vi "Test Remove.vi"() -> ()   [LabVIEW 2021, in "d15.lvlib" / "Cave.lvclass"]
uses:
  Cave.lvclass
  Diamond/Diamond.lvclass
panel:
  in  "Test":T1(ring)=enum."D in C"
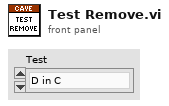
[diagram p1: front panel]
types:
  T1 = enum16{"D[1,2] in C", "D[1] in C", "D in C", "C[1,2] in D", "C in D", "D not in C"}
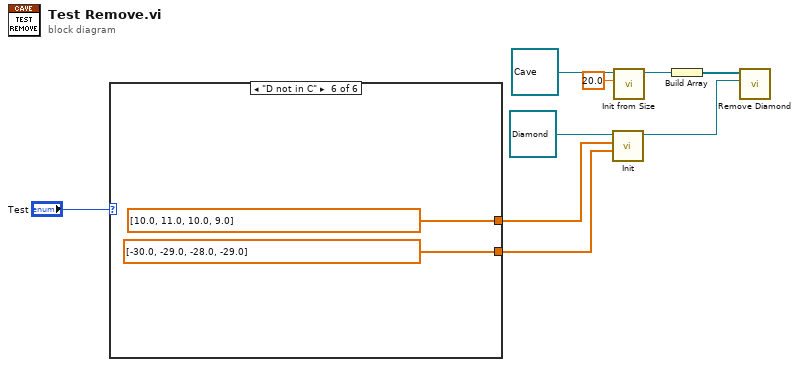
[diagram p0: block diagram]
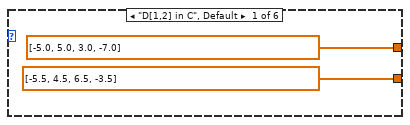
[diagram p2: hidden frame]
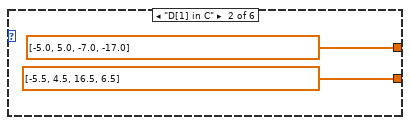
[diagram p3: hidden frame]
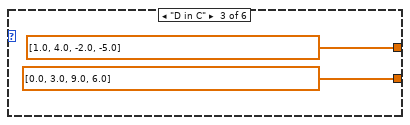
[diagram p4: hidden frame]
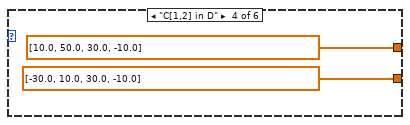
[diagram p5: hidden frame]
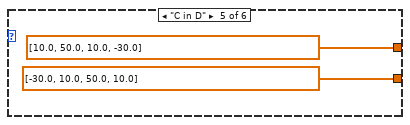
[diagram p6: hidden frame]
diagram:
  n1 = case shown="\"D not in C\"" "Test" {
    tunnel: [dbl[] [-5.0, 5.0, 3.0, -7.0] ("x") dbl[] [-5.0, 5.0, -7.0, -17.0] ("x") dbl[] [1.0, 4.0, -2.0, -5.0] ("x") dbl[] [10.0, 50.0, 30.0, -10.0] ("x") dbl[] [10.0, 50.0, 10.0, -30.0] ("x") dbl[] [10.0, 11.0, 10.0, 9.0] ("x")] -> w3
    tunnel: [dbl[] [-5.5, 4.5, 6.5, -3.5] ("y") dbl[] [-5.5, 4.5, 16.5, 6.5] ("y") dbl[] [0.0, 3.0, 9.0, 6.0] ("y") dbl[] [-30.0, 10.0, 30.0, -10.0] ("y") dbl[] [-30.0, 10.0, 50.0, 10.0] ("y") dbl[] [-30.0, -29.0, -28.0, -29.0] ("y")] -> w2
    frame "D[1,2] in C", Default {
    }
    frame "D[1] in C" {
    }
    frame "D in C" {
    }
    frame "C[1,2] in D" {
    }
    frame "C in D" {
    }
    frame "D not in C" {
    }
  }
  n2 = call-dynamic "Init.vi"("y"=w2, "x"=w3, "Diamond in"=refnum<class "Diamond.lvclass"> refnum ("d15.lvlib:Diamond.lvclass")) -> ("Diamond out"=w4:refnum<class "Diamond.lvclass">)  [unwired: 7 in, 1 out]
  n3 = call-dynamic "Init from Size.vi"("size"=20.0, "Cave  in"=refnum<class "Cave.lvclass"> refnum ("Caves in")) -> ("Cave out"=w7:refnum<class "Cave.lvclass">)  [unwired: 8 in, 1 out]
  n4 = Build Array(w7) -> (w9:refnum<class "Cave.lvclass">[])
  n5 = call "Remove Diamond.vi"("Diamond to Remove"=w4, "Caves in"=w9) -> ()  [unwired: 8 in, 2 out]
